vi "Simple Exception And Error Handler.vi"(11 "error in (no error)":errorcluster) -> (15 "error out":errorcluster)   [LabVIEW 2015, in "LV Exceptions v1.lvlib"]
uses:
  LV Exceptions v1.lvlib
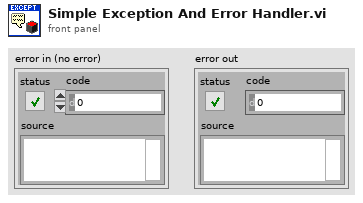
[diagram p1: front panel]
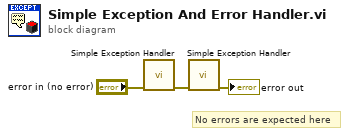
[diagram p0: block diagram]
diagram:
  # "No errors are expected here"
  n1 = call "Simple Exception Handler.vi"("error in (no error)"="error in (no error)") -> ("error out"=w2:errorcluster)  [unwired: 14 in]
  n2 = call "Simple Exception Handler.vi"("error in (no error)"=w2) -> ("error out"=→"error out":errorcluster)  [unwired: 14 in]
